vi "PulseGen.vi"(9 "CyclesPerMillisecond":u16, 10 "Pulse Generator Settings 1":T1={"Pulse Duration (ms)"=2, "Pulse Delay (ms)"=0, "Min Pulse Interval (ms)"=10}, 11 "Trigger":bool) -> (2 "PulseBufferOverflow":bool, 3 "PulseOut":bool)   [LabVIEW 2014]
panel:
  # "Pulse Settings"
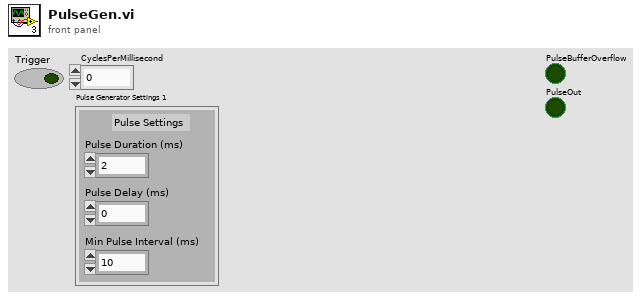
[diagram p1: front panel]
types:
  T1 = cluster{"Pulse Duration (ms)":u32, "Pulse Delay (ms)":u32, "Min Pulse Interval (ms)":u16}
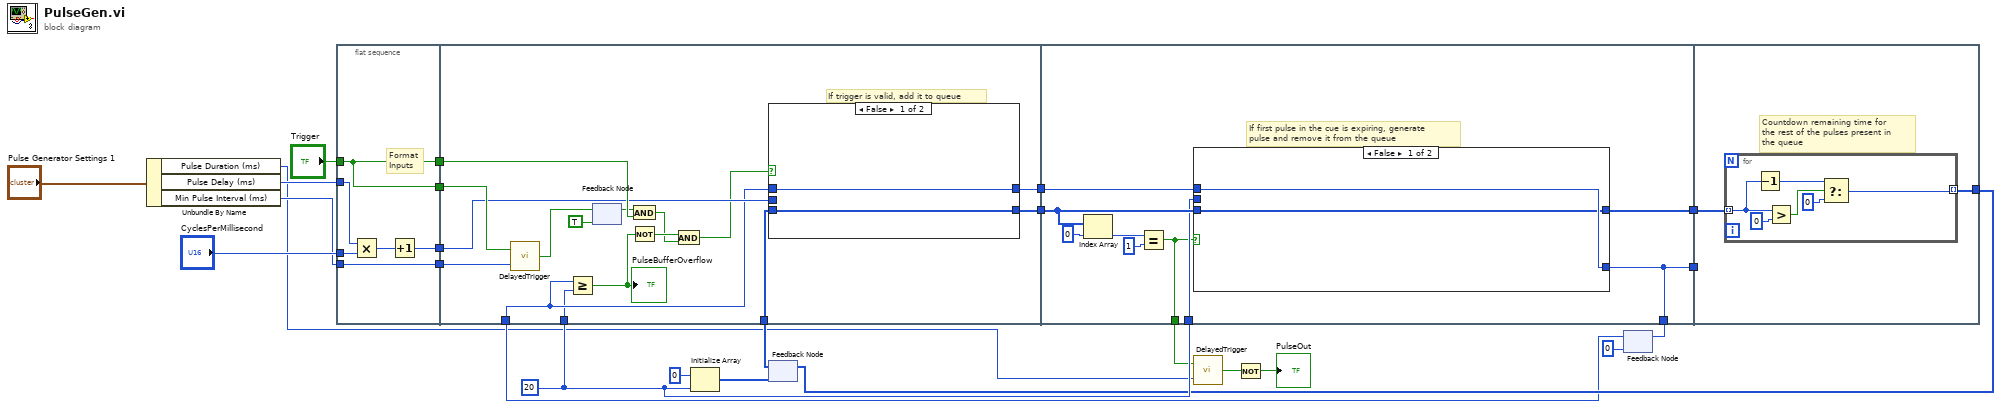
[diagram p0: block diagram]
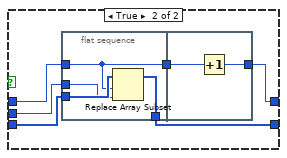
[diagram p2: hidden frame]
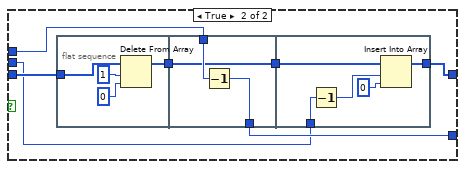
[diagram p3: hidden frame]
diagram:
  w23 = 20 ("dimension size")
  n1 = Unbundle By Name("Pulse Generator Settings 1") -> ("Pulse Duration (ms)"=w2:u32, "Pulse Delay (ms)"=w6:u32, "Min Pulse Interval (ms)"=w7:u16)
  n2 = flat-sequence {
    tunnel: [w26] -> w21
    tunnel: [w26] -> w20
    tunnel: [w31] -> w19
    tunnel: [w28] -> w18
    tunnel: "CyclesPerMillisecond" -> [w30]
    tunnel: w7 -> [w28]
    tunnel: w6 -> [w27]
    tunnel: "Trigger" -> [w26]
    tunnel: w21 -> [w47]
    tunnel: w20 -> [w46]
    tunnel: w12 -> [w45]
    tunnel: w9 -> [w43]
    tunnel: w19 -> [w44]
    tunnel: w23 -> [w42]
    tunnel: [w37] -> w17
    tunnel: [w36] -> w16
    tunnel: w18 -> [w35]
    tunnel: w17 -> [w67]
    tunnel: w16 -> [w66]
    tunnel: w23 -> [w65]
    tunnel: [w64] -> w15
    tunnel: [w63] -> w11
    tunnel: [w63] -> w14
    tunnel: [w62] -> w5
    tunnel: w15 -> [w93]
    tunnel: [w92] -> w13
    tunnel: w14 -> [_]
    frame #0 {
      # "Format\nInputs"
      n3 = Multiply(x=w27, y=w30) -> (x*y=w29:u32)
      n4 = Increment(x=w29) -> (x+1=w31:u32)
    }
    frame #1 {
      # "If trigger is valid, add it to queue"
      n5 = call "DelayedTrigger.vi"("Time Limit (ms)"=w35, "Initiate"=w47) -> ("Time Up"=w34:bool)
      n6 = Greater Or Equal?(x=w43, y=w42) -> (x >= y?=w41:bool)
      "PulseBufferOverflow" <- w41
      n7 = feedback-in #1(w34) -> ()
      n8 = feedback #1(TRUE ("Time Up")) -> (w33:bool)
      n9 = And(x=w33, y=w46) -> (x .and. y?=w39:bool)
      n10 = Not(x=w41) -> (.not. x?=w40:bool)
      n11 = And(x=w40, y=w39) -> (x .and. y?=w38:bool)
      n12 = case shown="False" w38 {
        tunnel: w45 -> [w48 w55]
        tunnel: w43 -> [w49 w54]
        tunnel: w44 -> [_ w53]
        tunnel: [w49 w51] -> w36
        tunnel: [w48 w50] -> w37
        frame False {
        }
        frame True {
          n13 = flat-sequence {
            tunnel: w55 -> [w59]
            tunnel: w54 -> [w57]
            tunnel: w53 -> [w56]
            tunnel: [w57] -> w52
            tunnel: [w58] -> w50
            tunnel: w52 -> [w61]
            tunnel: [w60] -> w51
            frame #0 {
              n14 = Replace Array Subset(array=w59, new element=w56, index=w57) -> (w58:u16[])
            }
            frame #1 {
              n15 = Increment(x=w61) -> (x+1=w60:u32)
            }
          }
        }
      }
    }
    frame #2 {
      # "If first pulse in the cue is expiring, generate \npulse and remove it from the queue"
      n16 = Index Array(array=w67, index=0) -> (element=w69:u16)
      n17 = Equal?(x=w69, y=u16 1) -> (x = y?=w62:bool)
      n18 = case shown="False" w62 {
        tunnel: w67 -> [w71 w79]
        tunnel: w66 -> [w72 w78]
        tunnel: [w72 w77] -> w63
        tunnel: w65 -> [_ w74]
        tunnel: [w71 w73] -> w64
        frame False {
        }
        frame True {
          n19 = flat-sequence {
            tunnel: w79 -> [w83]
            tunnel: [w80] -> w75
            tunnel: w78 -> [w86]
            tunnel: [w85] -> w77
            tunnel: [w84] -> w76
            tunnel: w75 -> [w84]
            tunnel: w76 -> [w91]
            tunnel: w74 -> [w90]
            tunnel: [w87] -> w73
            frame #0 {
              n20 = Delete From Array(array=w83, length=1, index=0) -> (array with subset deleted=w80:u16[])  [unwired: 1 out]
            }
            frame #1 {
              n21 = Decrement(x=w86) -> (x-1=w85:u32)
            }
            frame #2 {
              n22 = Decrement(x=w90) -> (x-1=w89:i32)
              n23 = Insert Into Array(array=w91, index=w89, new element=u16 0 ("new element/subarray")) -> (w87:u16[])
            }
          }
        }
      }
    }
    frame #3 {
      # "Countdown remaining time for\nthe rest of the pulses present in\nthe queue"
      n24 = for {
        tunnel: w93 -> [w97] mode=indexing
        tunnel: [w94] -> w92 mode=indexing
        n25 = Decrement(x=w97) -> (x-1=w96:u16)
        n26 = Greater?(x=w97, y=u16 0) -> (0:w98:bool)
        n27 = Select(t=w96, s=w98, f=u16 0) -> (s? t:f=w94:u16)
      }
    }
  }
  n28 = Initialize Array(u16 0, w23) -> (w24:u16[])
  n29 = feedback #2(w24) -> (w12:u16[])
  n30 = feedback-in #2(w13) -> ()
  n31 = call "DelayedTrigger.vi"("Time Limit (ms)"=w2, "Initiate"=w5) -> ("Time Up"=w4:bool)
  n32 = Not(x=w4) -> (.not. x?=→"PulseOut":bool)
  n33 = feedback #3(u32 0 ("index")) -> (w9:u32)
  n34 = feedback-in #3(w11) -> ()
